vi "GetCurrentCofiguration.vi"(8 "error in":errorcluster, 10 "Wanted configuration":T1=enum."VDC_AUTO", 11 "VISA resource name":refnum<visa-resource-name>) -> (0 "error out":errorcluster, 1 "Configuration Set":bool, 2 "Read data":string, 3 "VISA resource name out":refnum<visa-resource-name>)   [LabVIEW 2023, in "Aim TTi 1908P DMM.lvlib"]
uses:
  Aim TTi 1908P DMM.lvlib
  Configure.ctl
  a22fd55b-00fa-4424-8e5c-4af20e14b542.vi
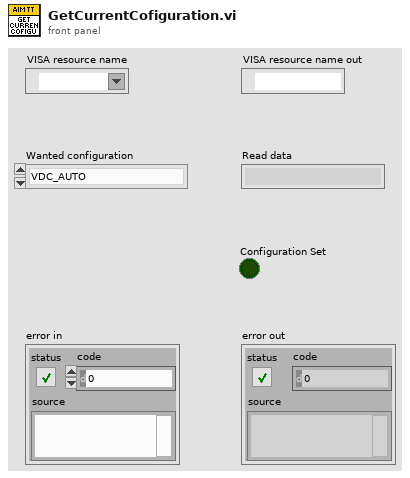
[diagram p1: front panel]
types:
  T1 = typedef "Aim TTi 1908P DMM.lvlib/Configure.ctl" = enum16{"VAC_750V", "VAC_100V", "VDC_AUTO", "VDC_100V", "VDC_1000mV", "VDC_100mV", "VDC_10V", "OHMS_AUTO", "OHMS_10K", "IDC_10A", "IDC_1mA", "IDC_100mA", "IDC_1000mA", "IAC_1mA", "IAC_100mA", "IAC_1000mA", "IAC_10A"}
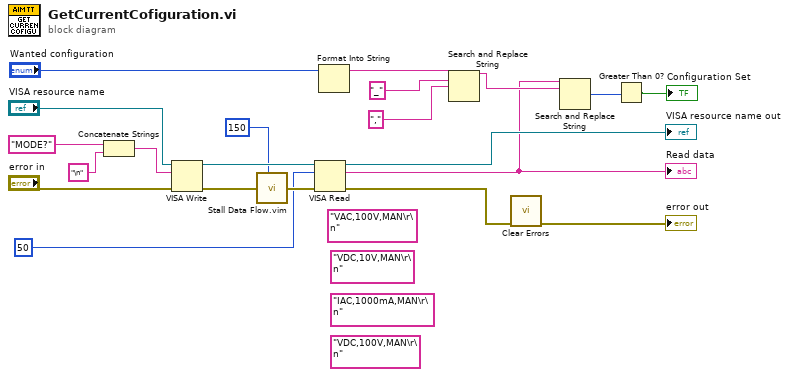
[diagram p0: block diagram]
diagram:
  (unwired) "IAC,1000mA,MAN\r\n" ("Read data 2")
  (unwired) "VDC,10V,MAN\r\n" ("Read data 2")
  (unwired) "VAC,100V,MAN\r\n" ("Read data 2")
  (unwired) "VDC,100V,MAN\r\n" ("Read data 2")
  n1 = Concatenate Strings("MODE?" ("Command"), "\n" ("string")) -> (w9:string)
  n2 = VISA Write(VISA resource name="VISA resource name", write buffer=w9, error in (no error)="error in") -> (VISA resource name out=w16:refnum<visa-resource-name>, error out=w15:errorcluster)  [unwired: 1 out]
  n3 = call "Stall Data Flow.vim"("value in"=w15, "milliseconds to wait"=u32 150) -> ("value out"=w14:errorcluster)  [unwired: 1 out]
  n4 = VISA Read(VISA resource name=w16, byte count=u32 50, error in (no error)=w14) -> (VISA resource name out=→"VISA resource name out":refnum<visa-resource-name>, read buffer=w3:string, error out=w6:errorcluster)  [unwired: 1 out]
  "Read data" <- w3
  n5 = Format Into String("Wanted configuration") -> (resulting string=w20:string)  [unwired: 3 in, 1 out]
  n6 = Search and Replace String(input string=w20, search string="_", replace string="," ("replace string (\"\")")) -> (result string=w17:string)  [unwired: 5 in, 3 out]
  n7 = call <vilib>:"Clear Errors.vi"("error in (no error)"=w6) -> ("error out"=→"error out":errorcluster)  [unwired: 5 in, 1 out]
  n8 = Search and Replace String(input string=w3, search string=w17) -> (number of replacements=w2:i32)  [unwired: 6 in, 3 out]
  n9 = Greater Than 0?(x=w2) -> (x > 0?=→"Configuration Set":bool)
